vi "Histogram2015.vi"() -> ()   [LabVIEW 2015]
uses:
  <vilib>/Analysis/NI_AALBase.lvlib
  <vilib>/Utility/file.llb/Read Delimited Spreadsheet (DBL).vi
panel:
  out "Prepared by \nthe project":string
  out "Data":dbl[][](array[numeric])
  out "Histogram":T1(graph)
  in  "Measurement file \nwith extension Txt":path
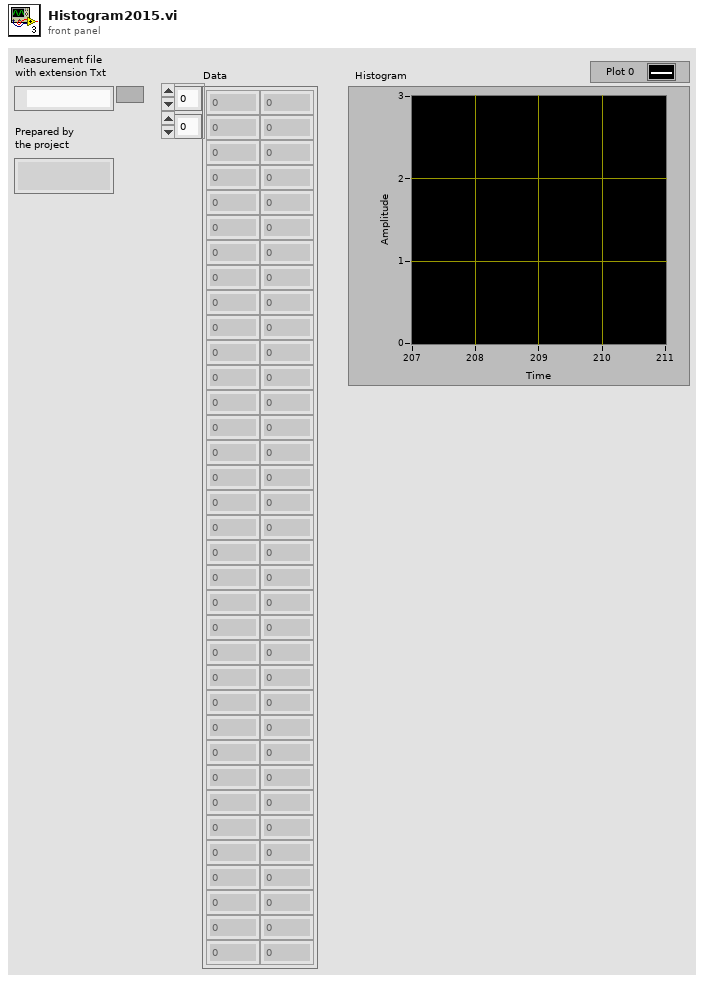
[diagram p1: front panel]
types:
  T1 = cluster{"X Values":dbl[], "Histogram: h(x)":i32[]}
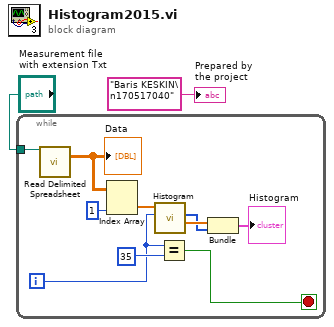
[diagram p0: block diagram]
diagram:
  n1 = while {
    tunnel: "Measurement file \nwith extension Txt" -> [w12]
    i -> [w3]
    stop <- w8 stop-if-true
    n2 = call-poly <vilib>:"Read Delimited Spreadsheet.vi"("file path (dialog if empty)"=w12) -> ("all rows"=w11:dbl[][])  [unwired: 9 in, 5 out]
    "Data" <- w11
    n3 = Index Array(array=w11, index (col)=1 ("disabled index (col)")) -> (element=w7:dbl[])  [unwired: 1 in]
    n4 = call <vilib>:"Histogram.vi"("intervals"=w3, "X"=w7) -> ("X Values"=w6:dbl[], "Histogram: h(x)"=w5:i32[])  [unwired: 6 in, 2 out]
    n5 = Equal?(x=w3, y=35) -> (x = y?=w8:bool)
    n6 = Bundle("X Values"=w6, "Histogram: h(x)"=w5) -> (→"Histogram":T1)  [unwired: 1 in]
  }
  "Prepared by \nthe project" <- "Baris KESKIN\n170517040"
